vi "PH_AxisGUI_6P.panel.vi"(0 "object ref":refnum<vi>, 5 "error in (no error)":errorcluster) -> (19 "error out":errorcluster)   [LabVIEW 2014, in "PH_AxisGUI_6P.lvlib"]
doc: "By this VI a ross relais can be monitored and switched. \n\nThe indicators \"CLOSED\", \"OPEN\" and \"SWITCH STATE\" show the value of the Beckhoff-Tag: blue indicates bad tag status reference problems, darkgreen false and lightgreen on. If everything is working fine, \"CLOSED\" and \"SWITCH STATE\" should show the same value, while \"OPEN\" has the opposite value. \n\nThe oval button switches the ross relais. It should be in the same state as the \"SWITCH STATE\" indicator. \n\n\"EXIT\" closes the front panel (GUI), while \"Delete Instance\" disconnects and removes the instance from the PCS.\n\nThis VI has no machine safety relevant logig: there is neither a check of internal conclict nor with other objects, for example conflict with other ross relais. Therefore it must be handled with care and should be operated by well educated operators only. It is forseen exclusively for direct operating and testing of the system. \n\nLicense Agreement for this software:\n\nCopyright (C)\nGesellschaft für Schwerionenforschung, GSI\nPlanckstr. 1\n64291 Darmstadt\nGermany\n\nContact: D.Beck@gsi.de \n\nThis program is free software; you can redistribute it and/or modify it under the terms of the GNU General Public License as published by the Free Software Foundation; either version 2 of the license, or (at your option) any later version.\n\nThis program is distributed in the hope that it will be useful, but WITHOUT ANYW ARRANTY; without even the implied warranty of MERCHANTABILITY or FITNESS FOR A PARTICULAR PURPOSE. See the GNU General License for more details (http://www.gnu.org).\n\nGesellschaft für Schwerionenforschung, GSI\nPlanckstr. 1, 64291 Darmstadt, Germany\nFor all questions and ideas contact: M.Richter@gsi.de, H.Brand@gsi.de or D.Beck@gsi.de.\nLast update: 18-DEC-2002"
uses:
  PH_AxisGUI_6P.lvlib
  PH_Stepmotor_BaseClass/PH_Stepmotor_BaseClass.Axis Settings.ctl
  PH_Stepmotor_BaseClass/PH_Stepmotor_BaseClass.Motor Type.ctl
  PH_Stepmotor_BaseClass/PH_Stepmotor_BaseClass.Axis Address.ctl
  PH_Stepmotor_BaseClass/PH_Stepmotor_BaseClass.Axis Activity.ctl
  PH_AxisGUI_BaseClass/PH_AxisGUI_BaseClass.Axis GUI Refs.ctl
  PH_Stepmotor_BaseClass/PH_Stepmotor_BaseClass.Axis Direction.ctl
  PH_Common/PH_Common.lvlib
  PH_AxisGUI_BaseClass/PH_AxisGUI_BaseClass.lvlib
  PH_Stepmotor_BaseClass/PH_Stepmotor_BaseClass.lvlib
  PH_Class/PH_Class.lvlib
panel:
  out "Activity Axis 2":T1
  out "Axis2_Status Bar":u32(colorbox) caption="Axis2"
  out "Axis2_Status":u32(colorbox)=6618880 caption="Axis2"
  out "Activity Axis 1":T1
  out "Axis1_Status Bar":u32(colorbox) caption="Axis1"
  out "Axis1_Status":u32(colorbox)=6618880 caption="Axis1"
  in  "Stop":bool caption="SetZero"
  in  "Tab Control":enum32{"Move", "Settings", "Info"}(tab)
  in  "Clear Error\nAxis 2":bool
  in  "Clear Error\nAxis 1":bool
  in  "DOWN":bool caption="? Steps"
  in  "UP":bool caption="? Steps"
  in  "LEFT":bool caption="? Steps"
  in  "RIGHT":bool caption="? Steps"
  in  "Axis2_Target":string="0" caption="Steps"
  in  "Axis1_Target":string="0" caption="Steps"
  in  "Axis2_Settings":T2={"Sign change"=FALSE, "Width"=0.0, "Calibration"=0.0, "Unit"="Steps", "Motor Type"=enum."Unspecific", "Unit Width"="", "Unit CF"=""} caption="Axis2"
  in  "Axis1_Settings":T2={"Sign change"=FALSE, "Width"=0.0, "Calibration"=0.0, "Unit"="Steps", "Motor Type"=enum."Unspecific", "Unit Width"="", "Unit CF"=""} caption="Axis1"
  in  "AxisSelection":enum32{"Axis1", "Axis2", "Both"}(radio)=enum."Both"
  in  "SetZero":bool
  in  "Reset":bool
  out "Address Axis 1":T4={"Instance"="N/A", "Motor Nr"=0} caption="Address Axis1"
  out "Address Axis 2":T4={"Instance"="N/A", "Motor Nr"=0} caption="Address Axis2"
  in  "Delete":bool
  # "PCS"
  # "3.40"
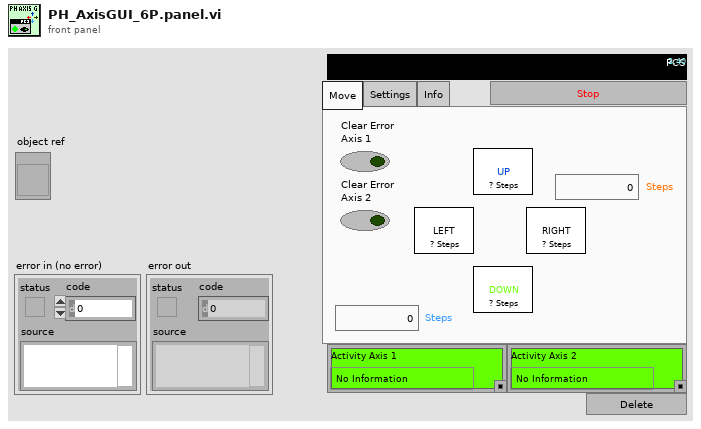
[diagram p1: front panel]
types:
  T1 = typedef "PH_Stepmotor_BaseClass.lvlib/PH_Stepmotor_BaseClass.Axis Activity.ctl" = enum16{"No Information", "stopped", "running", "Failure", "Alarm", "stopped at backward ES", "stopped at foreward ES"}
  T2 = typedef "PH_Stepmotor_BaseClass.lvlib/PH_Stepmotor_BaseClass.Axis Settings.ctl" = cluster{"Sign change":bool, "Width":dbl, "Calibration":dbl, "Unit":string, "Motor Type":T3, "Unit Width":string, "Unit CF":string}
  T3 = typedef "PH_Stepmotor_BaseClass.lvlib/PH_Stepmotor_BaseClass.Motor Type.ctl" = enum16{"Unspecific", "OWIS 49.120.2633", "OWIS 49.060.1033", "OWIS 43.040.2558", "Diamond Motion 2200 series", "OWIS 49.120.266B.MV6", "Calorimeter", "Linear Stage 1", "MICOS VT-80", "MICOS VT-80 S", "Standa Rotstage nt0.95A", "PUF RA 320.200", "PUF RA 800.200", "PUF RA 800.400", "PUF RA 400.50", "1324.nn.800.50", "1324.n9c.800.50", "1324.nn.320.200", "1324.nn.400.200", "1324.nn.800.200", "1324.nn.400.50", "1324.8c9c.800.50", "1324.8c9c.400.200"}
  T4 = typedef "PH_Stepmotor_BaseClass.lvlib/PH_Stepmotor_BaseClass.Axis Address.ctl" = cluster{"Instance":string, "Motor Nr":i32}
  T5 = typedef "PH_AxisGUI_BaseClass.lvlib/PH_AxisGUI_BaseClass.Axis GUI Refs.ctl" = cluster{"Back":refnum<vi>, "Forth":refnum<vi>, "Status":refnum<vi>, "Target":refnum<vi>, "Address":refnum<vi>, "Status Bar":refnum<vi>, "Settings":refnum<vi>, "Activity":refnum<vi>, "Clear Error":refnum<vi>}
  T6 = typedef "PH_Stepmotor_BaseClass.lvlib/PH_Stepmotor_BaseClass.Axis Direction.ctl" = enum16{"forward", "backward"}
  T7 = typedef "PH_AxisGUI_BaseClass.lvlib/PH_AxisGUI_BaseClass.i attribute.ctl" = cluster{"Axes":T8[]}
  T8 = typedef "PH_AxisGUI_BaseClass.lvlib/PH_AxisGUI_BaseClass.Axis Attributes.ctl" = cluster{"Axis GUI Refs":T5, "Address":T4, "Name":string, "Label \"Back\"":string, "Labell \"Forth\"":string, "Moving?":bool}
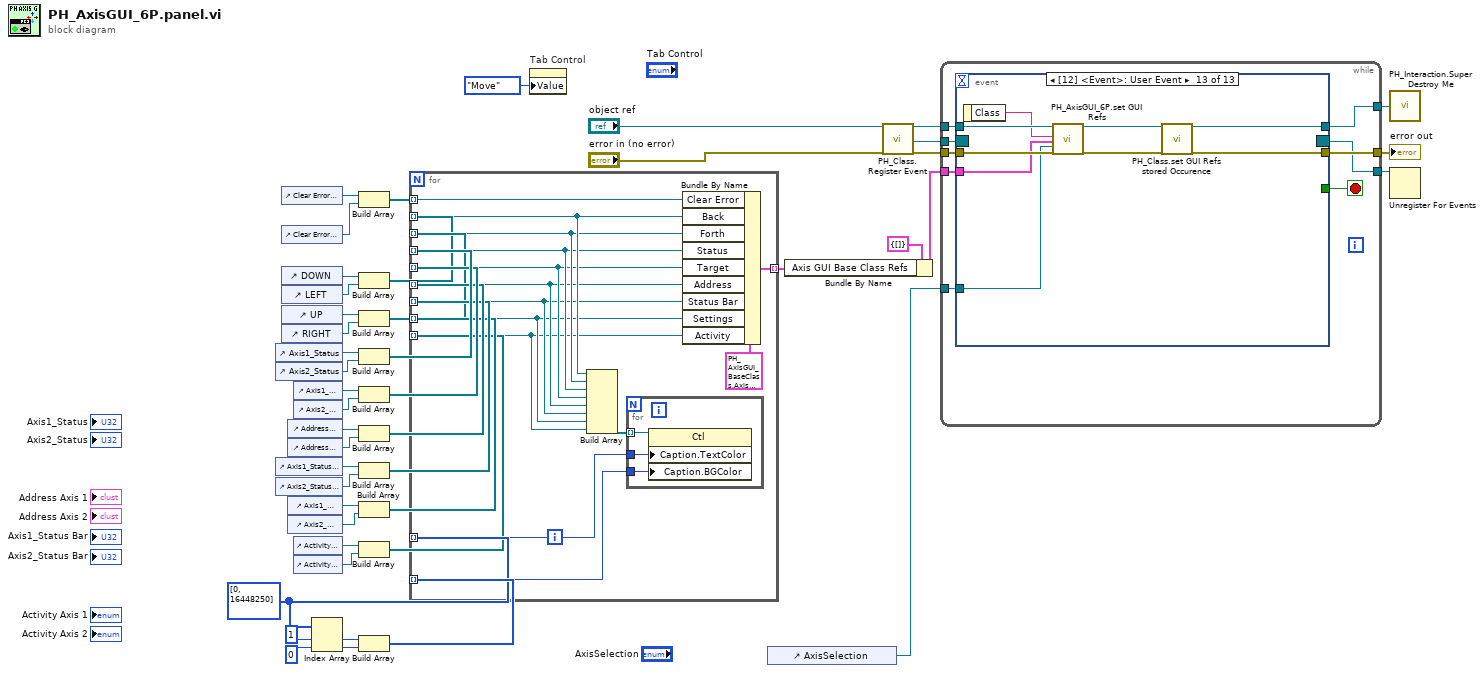
[diagram p0: block diagram]
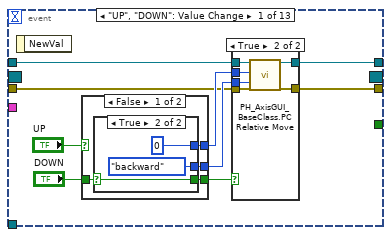
[diagram p2: hidden frame]
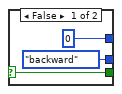
[diagram p3: hidden frame]
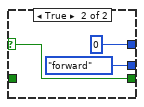
[diagram p4: hidden frame]
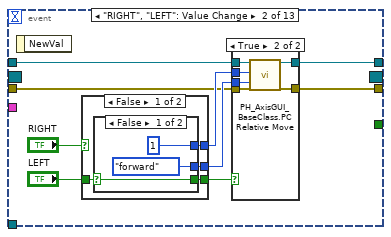
[diagram p6: hidden frame]
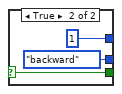
[diagram p7: hidden frame]
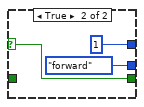
[diagram p8: hidden frame]
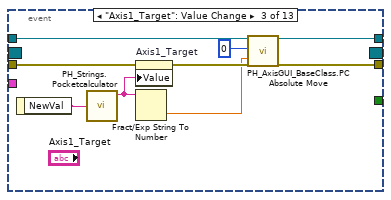
[diagram p10: hidden frame]
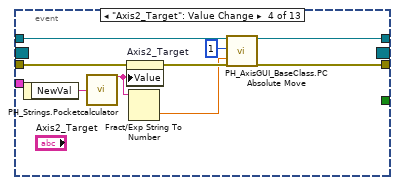
[diagram p11: hidden frame]
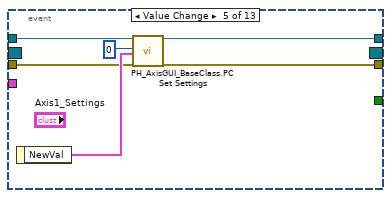
[diagram p12: hidden frame]
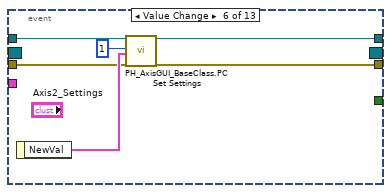
[diagram p13: hidden frame]
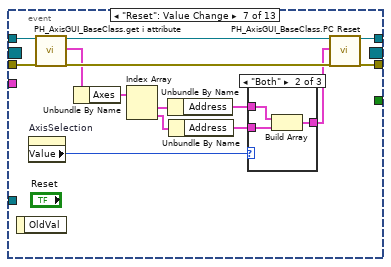
[diagram p14: hidden frame]
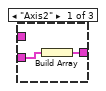
[diagram p15: hidden frame]
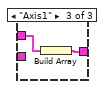
[diagram p16: hidden frame]
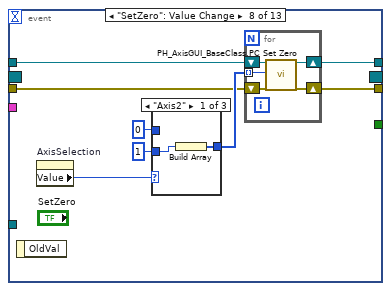
[diagram p17: hidden frame]
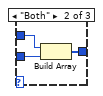
[diagram p18: hidden frame]
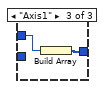
[diagram p19: hidden frame]
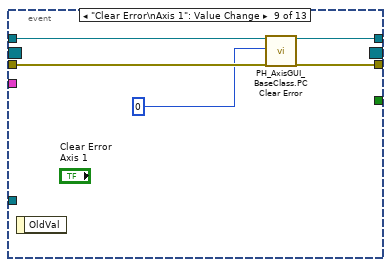
[diagram p20: hidden frame]
diagram:
  w22 = u32[] [0, 16448250]
  n1 = control-ref of="Axis1_Status"() -> (w40:refnum<vi>)
  n2 = control-ref of="Axis2_Status"() -> (w39:refnum<vi>)
  n3 = control-ref of="Axis1_Status Bar"() -> (w31:refnum<vi>)
  n4 = control-ref of="Axis2_Status Bar"() -> (w30:refnum<vi>)
  n5 = control-ref of="Clear Error\nAxis 1"() -> (w12:refnum<vi>)
  n6 = control-ref of="Clear Error\nAxis 2"() -> (w11:refnum<vi>)
  n7 = control-ref of="DOWN"() -> (w42:refnum<vi>)
  n8 = control-ref of="LEFT"() -> (w41:refnum<vi>)
  n9 = control-ref of="UP"() -> (w44:refnum<vi>)
  n10 = control-ref of="RIGHT"() -> (w43:refnum<vi>)
  n11 = control-ref of="Address Axis 1"() -> (w34:refnum<vi>)
  n12 = control-ref of="Address Axis 2"() -> (w33:refnum<vi>)
  n13 = control-ref of="Axis1_Settings"() -> (w19:refnum<vi>)
  n14 = control-ref of="Axis2_Settings"() -> (w18:refnum<vi>)
  n15 = control-ref of="Axis1_Target"() -> (w37:refnum<vi>)
  n16 = control-ref of="Axis2_Target"() -> (w36:refnum<vi>)
  n17 = control-ref of="Activity Axis 1"() -> (w21:refnum<vi>)
  n18 = control-ref of="Activity Axis 2"() -> (w20:refnum<vi>)
  n19 = Index Array(array=w22, index #1=1 ("index"), index #2=0 ("index")) -> (element #1=w25:u32, element #2=w24:u32)
  n20 = Build Array(w12, w11) -> (w13:refnum<vi>[])
  n21 = Build Array(w42, w41) -> (w16:refnum<vi>[])
  n22 = Build Array(w44, w43) -> (w17:refnum<vi>[])
  n23 = Build Array(w40, w39) -> (w38:refnum<vi>[])
  n24 = Build Array(w37, w36) -> (w35:refnum<vi>[])
  n25 = Build Array(w34, w33) -> (w32:refnum<vi>[])
  n26 = Build Array(w31, w30) -> (w29:refnum<vi>[])
  n27 = Build Array(w19, w18) -> (w28:refnum<vi>[])
  n28 = Build Array(w21, w20) -> (w15:refnum<vi>[])
  n29 = Build Array(w25, w24) -> (w23:u32[])
  n30 = for {
    tunnel: w16 -> [w58] mode=indexing
    tunnel: [w59] -> w5 mode=indexing
    tunnel: w17 -> [w57] mode=indexing
    tunnel: w38 -> [w56] mode=indexing
    tunnel: w35 -> [w55] mode=indexing
    tunnel: w32 -> [w54] mode=indexing
    tunnel: w29 -> [w53] mode=indexing
    tunnel: w28 -> [w52] mode=indexing
    tunnel: w15 -> [w48] mode=indexing
    tunnel: w23 -> [w50] mode=indexing
    tunnel: w22 -> [w49] mode=indexing
    tunnel: w13 -> [w47] mode=indexing
    n31 = Build Array(w58, w57, w56, w55, w54, w53, w52, w48) -> (w51:refnum<vi>[])
    n32 = for {
      tunnel: w51 -> [w63] mode=indexing
      tunnel: w50 -> [w62]
      tunnel: w49 -> [w61]
      n33 = property class="Ctl"(reference=w63, "Caption.TextColor"=w61, "Caption.BGColor"=w62) -> ()  [unwired: 1 in, 2 out]
    }
    n34 = Bundle By Name(cluster=T5 {"Back"=refnum, "Forth"=refnum, "Status"=refnum, "Target"=refnum, "Address"=refnum, "Status Bar"=refnum, "Settings"=refnum, "Activity"=refnum, "Clear Error"=refnum} ("GUI Refs"), "Clear Error"=w47, "Back"=w58, "Forth"=w57, "Status"=w56, "Target"=w55, "Address"=w54, "Status Bar"=w53, "Settings"=w52, "Activity"=w48) -> (w59:T5)
  }
  n35 = property on="Tab Control" class="TabCtl (strict)"("Value"=enum32{"Move", "Settings", "Info"}."Move" ("Tab Control")) -> ()  [unwired: 2 in, 2 out]
  n36 = control-ref of="AxisSelection"() -> (w1:refnum<vi>)
  n37 = Bundle By Name(cluster=cluster{"Axis GUI Base Class Refs":T5[]} {"Axis GUI Base Class Refs"=[]} ("GUI Refs"), "Axis GUI Base Class Refs"=w5) -> (w4:cluster{"Axis GUI Base Class Refs":T5[]})
  n38 = call "PH_Class.Register Event.vi"("i ref in"="object ref", "error in (no error)"="error in (no error)") -> ("i ref out"=w10:refnum<vi>, "Event Registration Refnum"=w8:refnum<event-registration>, "error out"=w9:errorcluster)  [unwired: 15 in]
  n39 = while {
    tunnel: w10 -> [w69]
    tunnel: [w68] -> w45
    tunnel: w9 -> [w71]
    tunnel: [w70] -> w46
    tunnel: w8 -> [w67]
    tunnel: [w66] -> w7
    tunnel: w4 -> [w65]
    tunnel: w1 -> [w64]
    stop <- w72 stop-if-true
    n40 = event shown="[12] <Event>: User Event" {
      selector: w67 -> [_ _ _ _ _ _ _ _ _ _ _ _ _]
      dyn-events: [_ _ _ _ _ _ _ _ _ _ _ _ _] -> w66
      timeout: _ -> [_ _ _ _ _ _ _ _ _ _ _ _ _]
      tunnel: [_ _ _ _ _ _ _ _ _ _ _ "Delete" _] -> w72
      tunnel: w69 -> [w78 w108 w135 w143 w152 w159 w173 w185 w206 w211 w215 w220 w231]
      tunnel: w71 -> [w76 w106 w134 w144 w151 w158 w171 w184 w205 w210 w214 w221 w230]
      tunnel: [w75 w105 w140 w149 w156 w162 w170 w190 w207 w212 w216 w218 w225] -> w70
      tunnel: [w77 w107 w139 w148 w155 w161 w172 w191 w208 w213 w217 w219 w223] -> w68
      tunnel: w65 -> [_ _ _ _ _ _ _ _ _ _ _ _ w227]
      tunnel: w64 -> [_ _ _ _ _ _ _ _ _ _ _ _ w226]
      event "UP", "DOWN": Value Change {
        n41 = event-data() -> ()  [unwired: 1 in, 1 out]
        n42 = case shown="False" "UP" {
          selector: "UP" -> [_ w92]
          tunnel: [w85 0] -> w80
          tunnel: [w84 PH_Stepmotor_BaseClass.Axis_Direction."forward" ("direction")] -> w81
          tunnel: "DOWN" -> [w83 _]
          tunnel: [w82 w92] -> w79
          frame False {
            n43 = case shown="True" w83 {
              selector: w83 -> [w86 w89]
              tunnel: [0 0] -> w85
              tunnel: [PH_Stepmotor_BaseClass.Axis_Direction."backward" ("direction") PH_Stepmotor_BaseClass.Axis_Direction."backward" ("direction")] -> w84
              tunnel: [w86 w89] -> w82
              frame False {
              }
              frame True {
              }
            }
          }
          frame True {
          }
        }
        n44 = case shown="True" w79 {
          tunnel: w76 -> [w95 w102]
          tunnel: w78 -> [w96 w101]
          tunnel: w81 -> [_ w100]
          tunnel: [w96 w99] -> w77
          tunnel: [w95 w98] -> w75
          tunnel: w80 -> [_ w97]
          frame False {
          }
          frame True {
            n45 = call "PH_AxisGUI_BaseClass.PC Relative Move.vi"("i ref in"=w101, "Axis"=w97, "direction"=w100, "error in"=w102) -> ("i ref out"=w99:refnum<vi>, "error out"=w98:errorcluster)  [unwired: 14 in]
          }
        }
      }
      event "RIGHT", "LEFT": Value Change {
        n46 = event-data() -> ()  [unwired: 1 in, 1 out]
        n47 = case shown="False" "RIGHT" {
          selector: "RIGHT" -> [_ w122]
          tunnel: [w115 1] -> w110
          tunnel: [w114 PH_Stepmotor_BaseClass.Axis_Direction."forward" ("direction")] -> w111
          tunnel: "LEFT" -> [w113 _]
          tunnel: [w112 w122] -> w109
          frame False {
            n48 = case shown="False" w113 {
              selector: w113 -> [w116 w119]
              tunnel: [1 1] -> w115
              tunnel: [PH_Stepmotor_BaseClass.Axis_Direction."forward" ("direction") PH_Stepmotor_BaseClass.Axis_Direction."backward" ("direction")] -> w114
              tunnel: [w116 w119] -> w112
              frame False {
              }
              frame True {
              }
            }
          }
          frame True {
          }
        }
        n49 = case shown="True" w109 {
          tunnel: w106 -> [w125 w132]
          tunnel: w108 -> [w126 w131]
          tunnel: w111 -> [_ w130]
          tunnel: [w126 w129] -> w107
          tunnel: [w125 w128] -> w105
          tunnel: w110 -> [_ w127]
          frame False {
          }
          frame True {
            n50 = call "PH_AxisGUI_BaseClass.PC Relative Move.vi"("i ref in"=w131, "Axis"=w127, "direction"=w130, "error in"=w132) -> ("i ref out"=w129:refnum<vi>, "error out"=w128:errorcluster)  [unwired: 14 in]
          }
        }
      }
      event "Axis1_Target": Value Change {
        n51 = event-data() -> ("NewVal"=w141:string)  [unwired: 1 in]
        n52 = call "PH_Strings.Pocketcalculator.vi"("Input"=w141) -> ("String Double"=w138:string)  [unwired: 3 out]
        n53 = property on="Axis1_Target" class="Str"(error in=w134, "Value"=w138) -> (error out=w137:errorcluster)  [unwired: 1 in, 1 out]
        n54 = Fract/Exp String To Number(string=w138) -> (number=w136:dbl)  [unwired: 3 in, 1 out]
        n55 = call "PH_AxisGUI_BaseClass.PC Absolute Move.vi"("i ref in"=w135, "Axis"=0, "Position [Units]"=w136, "error in"=w137) -> ("i ref out"=w139:refnum<vi>, "error out"=w140:errorcluster)  [unwired: 14 in]
      }
      event "Axis2_Target": Value Change {
        n56 = event-data() -> ("NewVal"=w150:string)  [unwired: 1 in]
        n57 = call "PH_Strings.Pocketcalculator.vi"("Input"=w150) -> ("String Double"=w147:string)  [unwired: 3 out]
        n58 = property on="Axis2_Target" class="Str"(error in=w144, "Value"=w147) -> (error out=w146:errorcluster)  [unwired: 1 in, 1 out]
        n59 = Fract/Exp String To Number(string=w147) -> (number=w145:dbl)  [unwired: 3 in, 1 out]
        n60 = call "PH_AxisGUI_BaseClass.PC Absolute Move.vi"("i ref in"=w143, "Axis"=1, "Position [Units]"=w145, "error in"=w146) -> ("i ref out"=w148:refnum<vi>, "error out"=w149:errorcluster)  [unwired: 14 in]
      }
      event Value Change {
        n61 = event-data() -> ("NewVal"=w154:T2)  [unwired: 1 in]
        n62 = call "PH_AxisGUI_BaseClass.PC Set Settings.vi"("VI in"=w152, "Axis"=0, "NewVal"=w154, "error in (no error)"=w151) -> ("VI out"=w155:refnum<vi>, "error out"=w156:errorcluster)  [unwired: 14 in]
      }
      event Value Change {
        n63 = event-data() -> ("NewVal"=w160:T2)  [unwired: 1 in]
        n64 = call "PH_AxisGUI_BaseClass.PC Set Settings.vi"("VI in"=w159, "Axis"=1, "NewVal"=w160, "error in (no error)"=w158) -> ("VI out"=w161:refnum<vi>, "error out"=w162:errorcluster)  [unwired: 14 in]
      }
      event "Reset": Value Change {
        n65 = event-data() -> ()  [unwired: 1 in, 1 out]
        n66 = property on="AxisSelection" class="RadioBtnsControl (strict)"() -> ("Value"=w169:enum32{"Axis1", "Axis2", "Both"})  [unwired: 2 in, 2 out]
        n67 = call "PH_AxisGUI_BaseClass.get i attribute.vi"("i ref in"=w173, "error in (no error)"=w171) -> ("i ref out"=w175:refnum<vi>, "i attribute"=w168:T7, "error out"=w176:errorcluster)  [unwired: 15 in]
        n68 = Unbundle By Name(w168) -> ("Axes"=w167:T8[])
        n69 = Index Array(array=w167) -> (element #1=w166:T8, element #2=w165:T8)  [unwired: 2 in]
        n70 = Unbundle By Name(w166) -> ("Address"=w163:T4)
        n71 = Unbundle By Name(w165) -> ("Address"=w164:T4)
        n72 = case shown="\"Both\"" w169 {
          tunnel: [w178 w181 w183] -> w174
          tunnel: w164 -> [w177 w180 _]
          tunnel: w163 -> [_ w179 w182]
          frame "Axis2" {
            n73 = Build Array(w177) -> (w178:T4[])
          }
          frame "Both" {
            n74 = Build Array(w179, w180) -> (w181:T4[])
          }
          frame "Axis1" {
            n75 = Build Array(w182) -> (w183:T4[])
          }
        }
        n76 = call "PH_AxisGUI_BaseClass.PC Reset.vi"("i ref in"=w175, "Addresses"=w174, "error in"=w176) -> ("i ref out"=w172:refnum<vi>, "error out"=w170:errorcluster)  [unwired: 15 in]
      }
      event "SetZero": Value Change {
        n77 = event-data() -> ()  [unwired: 1 in, 1 out]
        n78 = property on="AxisSelection" class="RadioBtnsControl (strict)"() -> ("Value"=w189:enum32{"Axis1", "Axis2", "Both"})  [unwired: 2 in, 2 out]
        n79 = case shown="\"Axis2\"" w189 {
          tunnel: [w198 w201 w203] -> w188
          tunnel: 1 -> [w197 w200 _]
          tunnel: 0 -> [_ w199 w202]
          frame "Axis2" {
            n80 = Build Array(w197) -> (w198:i32[])
          }
          frame "Both" {
            n81 = Build Array(w199, w200) -> (w201:i32[])
          }
          frame "Axis1" {
            n82 = Build Array(w202) -> (w203:i32[])
          }
        }
        n83 = for {
          tunnel: w188 -> [w192] mode=indexing
          shift-right: [w193] -> w190
          shift-left: w184 -> [w196]
          shift-right: [w194] -> w191
          shift-left: w185 -> [w195]
          n84 = call "PH_AxisGUI_BaseClass.PC Set Zero.vi"("VI in"=w195, "Axis"=w192, "error in (no error)"=w196) -> ("VI out"=w194:refnum<vi>, "error out"=w193:errorcluster)  [unwired: 15 in]
        }
      }
      event "Clear Error\nAxis 1": Value Change {
        n85 = event-data() -> ()  [unwired: 1 in, 1 out]
        n86 = call "PH_AxisGUI_BaseClass.PC Clear Error.vi"("i ref in"=w206, "Axis"=0, "error in"=w205) -> ("i ref out"=w208:refnum<vi>, "error out"=w207:errorcluster)  [unwired: 15 in]
      }
      event "Clear Error\nAxis 2": Value Change {
        n87 = event-data() -> ()  [unwired: 1 in, 1 out]
        n88 = call "PH_AxisGUI_BaseClass.PC Clear Error.vi"("i ref in"=w211, "Axis"=1, "error in"=w210) -> ("i ref out"=w213:refnum<vi>, "error out"=w212:errorcluster)  [unwired: 15 in]
      }
      event "Stop": Value Change {
        n89 = event-data() -> ()  [unwired: 1 in, 2 out]
        n90 = call "PH_AxisGUI_BaseClass.PC Stop.vi"("VI in"=w215, "error in (no error)"=w214) -> ("VI out"=w217:refnum<vi>, "error out"=w216:errorcluster)  [unwired: 16 in]
      }
      event "Delete": Value Change {
        n91 = event-data() -> ()  [unwired: 1 in, 1 out]
        n92 = call "PH_Class.Delete GUI.vi"("VI in"=w220, "error in (no error)"=w221) -> ("VI out"=w219:refnum<vi>, "error out"=w218:errorcluster)  [unwired: 16 in]
      }
      event User Event {
        n93 = event-data() -> ("Class"=w228:string)  [unwired: 1 in]
        n94 = call "PH_AxisGUI_6P.set GUI Refs.vi"("i ref in"=w231, "Class"=w228, "GUI Refs"=w227, "AxisSelection"=w226, "error in"=w230) -> ("i ref out"=w224:refnum<vi>, "error out"=w229:errorcluster)  [unwired: 13 in]
        n95 = call "PH_Class.set GUI Refs stored Occurence.vi"("i ref in"=w224, "error in (no error)"=w229) -> ("i ref out"=w223:refnum<vi>, "error out"=w225:errorcluster)  [unwired: 16 in]
      }
    }
  }
  "error out" <- w46
  n96 = call "PH_Interaction.Super Destroy Me.vi"("i ref out"=w45) -> ()
  n97 = Unregister For Events(event registration refnum=w7) -> ()  [unwired: 1 in, 1 out]
